vi "NicmosSetReadNumber.vi"(1 "Read Number":i32=2, 2 "Degitch":i32, 8 "error in":errorcluster caption="entrée d'erreur") -> (5 "error out":errorcluster caption="sortie d'erreur")   [LabVIEW 2009]
doc: "Définition du nombre de lecture du détecteur, de la vitesse de lecture, du mode de lecture et réservation du buffer de lecture associé."
uses:
  NicmosGlobal.vi
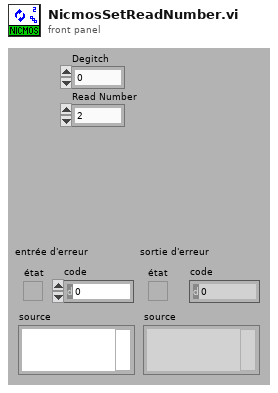
[diagram p1: front panel]
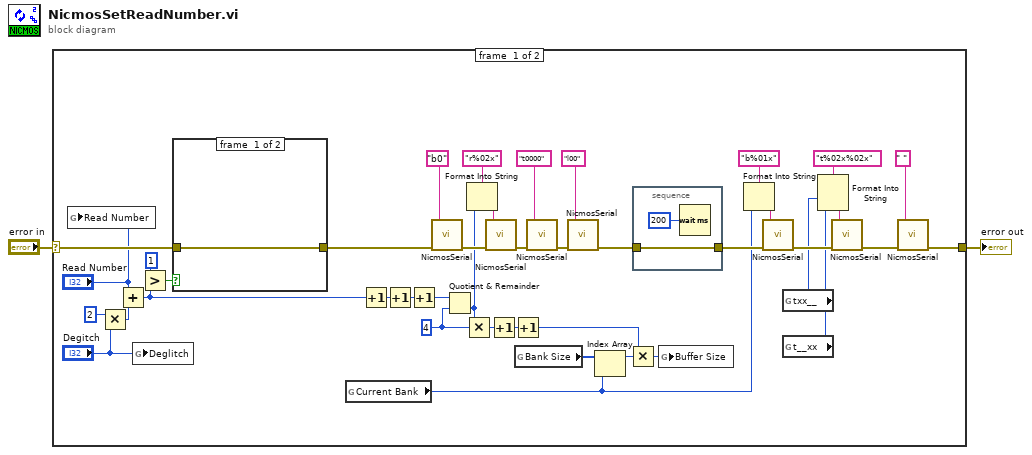
[diagram p0: block diagram]
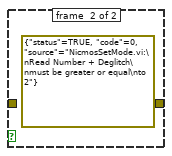
[diagram p2: hidden frame]
diagram:
  n1 = case shown="No Error" "error in" {
    selector: "error in" -> [w40 w48]
    tunnel: [w4 w48] -> w2
    frame #0 {
      w21 = 4 ("y")
      n2 = global write "NicmosGlobal.vi" "Read Number"("Read Number") -> ()
      n3 = Multiply(x=2, y="Degitch") -> (x*y=w30:i32)
      n4 = Add(x="Read Number", y=w30) -> (x+y=w7:i32)
      n5 = global write "NicmosGlobal.vi" "Deglitch"("Degitch") -> ()
      n6 = Greater?(x=1 ("y"), y=w7) -> (0:w42:bool)
      n7 = case shown="False" w42 {
        tunnel: w40 -> [w46 _]
        tunnel: [w46 errorcluster {"status"=TRUE, "code"=0, "source"="NicmosSetMode.vi:\nRead Number + Deglitch\nmust be greater or equal\nto 2"} ("error in")] -> w41
        frame #0 {
        }
        frame #1 {
        }
      }
      n8 = global read "NicmosGlobal.vi" "Current Bank"() -> (w36:i32)
      n9 = Increment(x=w7) -> (x+1=w14:i32)
      n10 = Increment(x=w14) -> (x+1=w15:i32)
      n11 = Increment(x=w15) -> (x+1=w20:i32)
      n12 = call "NicmosSerial.vi"("error in"=w41, "Command"="b0") -> ("error out"=w24:errorcluster)  [unwired: 3 in, 1 out]
      n13 = Quotient & Remainder(x=w20, y=w21) -> (floor(x/y)=w11:i32)  [unwired: 1 out]
      n14 = Multiply(x=w21, y=w11) -> (x*y=w19:i32)
      n15 = Format Into String(format string="r%02x" ("Question L"), w11) -> (resulting string=w27:string)  [unwired: 2 in, 1 out]
      n16 = call "NicmosSerial.vi"("error in"=w24, "Command"=w27) -> ("error out"=w22:errorcluster)  [unwired: 3 in, 1 out]
      n17 = Increment(x=w19) -> (x+1=w18:i32)
      n18 = Increment(x=w18) -> (x+1=w12:i32)
      n19 = global read "NicmosGlobal.vi" "Bank Size"() -> (w16:i32[])
      n20 = call "NicmosSerial.vi"("error in"=w22, "Command"="t0000") -> ("error out"=w9:errorcluster)  [unwired: 3 in, 1 out]
      n21 = call "NicmosSerial.vi"("error in"=w9, "Command"="l00") -> ("error out"=w8:errorcluster)  [unwired: 3 in, 1 out]
      n22 = Index Array(array=w16, index=w36) -> (element=w13:i32)
      n23 = Multiply(x=w13, y=w12) -> (x*y=w17:i32)
      n24 = stacked-sequence {
        tunnel: w8 -> [w45]
        tunnel: [w45] -> w37
        frame #0 {
          n25 = Wait (ms)(milliseconds to wait=u32 200 ("attente (ms)")) -> ()  [unwired: 1 out]
        }
      }
      n26 = global write "NicmosGlobal.vi" "Buffer Size"(w17) -> ()
      n27 = Format Into String(format string="b%01x" ("Chaîne d'entrée"), w36) -> (resulting string=w39:string)  [unwired: 2 in, 1 out]
      n28 = call "NicmosSerial.vi"("error in"=w37, "Command"=w39) -> ("error out"=w33:errorcluster)  [unwired: 3 in, 1 out]
      n29 = global read "NicmosGlobal.vi" "txx__"() -> (w32:i32)
      n30 = global read "NicmosGlobal.vi" "t__xx"() -> (w31:i32)
      n31 = Format Into String(format string="t%02x%02x" ("Question L"), w32, w31) -> (resulting string=w35:string)  [unwired: 2 in, 1 out]
      n32 = call "NicmosSerial.vi"("error in"=w33, "Command"=w35) -> ("error out"=w5:errorcluster)  [unwired: 3 in, 1 out]
      n33 = call "NicmosSerial.vi"("error in"=w5, "Command"=" ") -> ("error out"=w4:errorcluster)  [unwired: 3 in, 1 out]
    }
    frame #1 {
    }
  }
  "error out" <- w2
